vi "Perform Step.vi"(8 "error in (no error)":errorcluster, 11 "Mouse Macro in":refnum<class "Mouse Macro.lvclass">) -> (0 "error out":errorcluster, 2 "Result":T1, 3 "Mouse Macro out":refnum<class "Mouse Macro.lvclass">)   [LabVIEW 2023, in "MacroAssert.lvlib" / "Mouse Macro.lvclass"]
uses:
  Mouse Macro.lvclass
  Mouse Macro.lvclass/Mouse Macro.ctl
  MacroAssert.lvlib
  ca4cad37-3336-401d-b470-0dddd82eef88.vi
  CTLs/Report Data.ctl
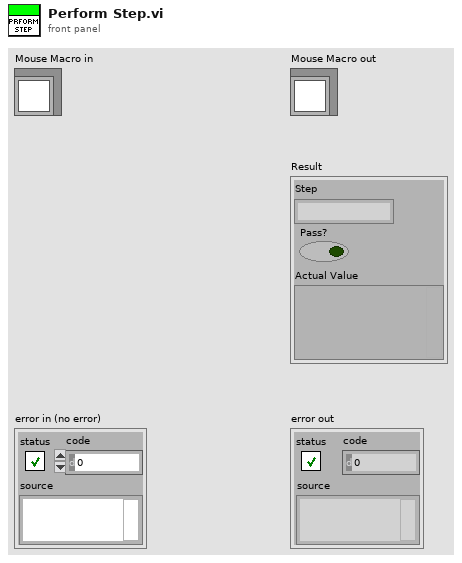
[diagram p1: front panel]
types:
  T1 = typedef "MacroAssert.lvlib/Report Data.ctl" = cluster{"Step":string, "Pass?":bool, "Actual Value":variant}
  T2 = typedef "MacroAssert.lvlib/Step Type V3.ctl" = enum16{"Mouse Move", "Mouse Click", "Key Press", "Wait", "Mouse Down", "Mouse Up", "Key Down", "Key Up", "Test Assertion", "Maximize Window", "Restore Window", "Minimize Window", "Close Window", "Bring Window to Front", "Send Window to Back"}
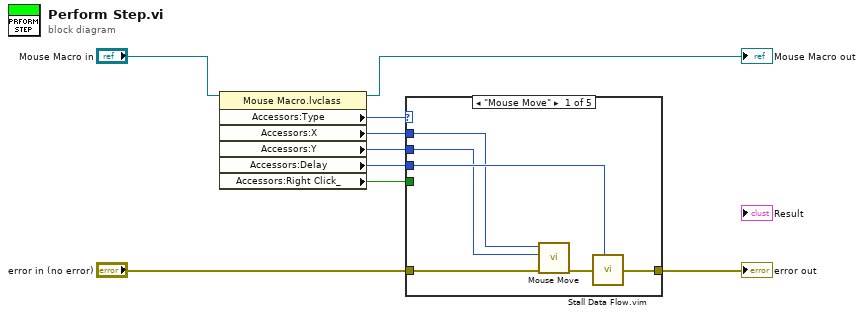
[diagram p0: block diagram]
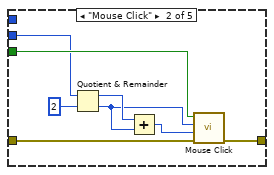
[diagram p2: hidden frame]
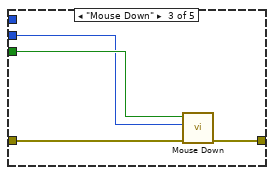
[diagram p3: hidden frame]
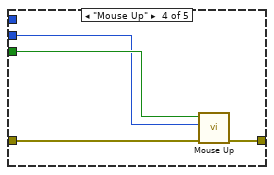
[diagram p4: hidden frame]
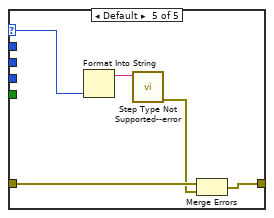
[diagram p5: hidden frame]
diagram:
  n1 = property class="Mouse Macro.lvclass"(reference="Mouse Macro in") -> (reference out=→"Mouse Macro out":refnum<class "Mouse Macro.lvclass">, "Accessors:Type"=w5:T2, "Accessors:X"=w4:i32, "Accessors:Y"=w3:i32, "Accessors:Delay"=w2:i32, "Accessors:Right Click_"=w1:bool)  [unwired: 1 in, 1 out]
  n2 = case shown="\"Mouse Move\"" w5 {
    selector: w5 -> [_ _ _ _ w36]
    tunnel: w4 -> [w12 _ _ _ _]
    tunnel: w2 -> [w13 w21 w25 w29 _]
    tunnel: [w14 w23 w27 w31 w32] -> w8
    tunnel: w1 -> [_ w22 w26 w30 _]
    tunnel: w3 -> [w11 _ _ _ _]
    tunnel: "error in (no error)" -> [w10 w16 w24 w28 w34]
    frame "Mouse Move" {
      n3 = call "Mouse Move.vi"("error in (no error)"=w10, "y"=w11, "x"=w12) -> ("error out"=w15:errorcluster)  [unwired: 8 in]
      n4 = call "Stall Data Flow.vim"("value in"=w15, "milliseconds to wait"=w13) -> ("value out"=w14:errorcluster)  [unwired: 1 out]
    }
    frame "Mouse Click" {
      n5 = Quotient & Remainder(x=w21, y=2) -> (x-y*floor(x/y)=w19:i32, floor(x/y)=w17:i32)
      n6 = Add(x=w19, y=w17) -> (x+y=w18:i32)
      n7 = call "Mouse Click.vi"("error in (no error)"=w16, "ms wait after up (10)"=w18, "ms wait after down (10)"=w17, "Right Click? (F)"=w22) -> ("error out"=w23:errorcluster)  [unwired: 7 in]
    }
    frame "Mouse Down" {
      n8 = call "Mouse Down.vi"("error in (no error)"=w24, "Delay in ms (10)"=w25, "Right Click? (F)"=w26) -> ("error out"=w27:errorcluster)  [unwired: 8 in]
    }
    frame "Mouse Up" {
      n9 = call "Mouse Up.vi"("error in (no error)"=w28, "Delay in ms (10)"=w29, "Right Click? (F)"=w30) -> ("error out"=w31:errorcluster)  [unwired: 8 in]
    }
    frame Default {
      n10 = Format Into String(w36) -> (resulting string=w35:string)  [unwired: 3 in, 1 out]
      n11 = call "Step Type Not Supported--error.vi"("Step Type"=w35) -> ("error out"=w33:errorcluster)  [unwired: 10 in]
      n12 = Merge Errors(w34, w33) -> (w32:errorcluster)
    }
  }
  "error out" <- w8
